vi "MeasurementItems_GetTransferNumber.vi"(8 "error in (no error)":errorcluster, 11 "OXY_SCPI Reseource In":refnum<visa-resource-name>) -> (0 "error out":errorcluster, 1 "communication_data":T1, 2 "Num Transfer Items":i32, 3 "OXY_SCPI Reseource Out":refnum<visa-resource-name>)   [LabVIEW 2018, in "OXYGEN.lvlib"]
doc: "Queries the number of items to be transferred."
uses:
  OXYGEN.lvlib
  TypeDefs/Cluster_RawCommData.ctl
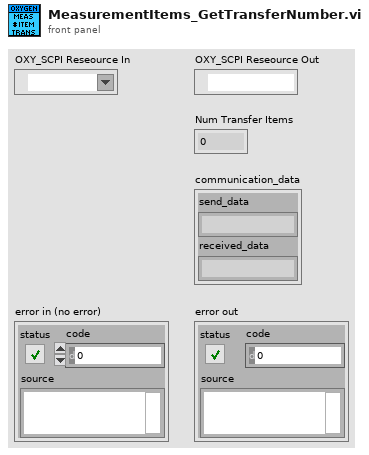
[diagram p1: front panel]
types:
  T1 = typedef "OXYGEN.lvlib/Cluster_RawCommData.ctl" = cluster{"send_data":string, "received_data":string}
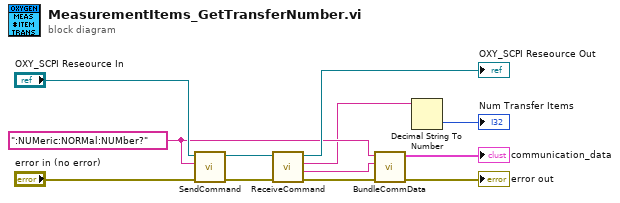
[diagram p0: block diagram]
diagram:
  w4 = ":NUMeric:NORMal:NUMber?" ("String to Send")
  n1 = call "SendCommand.vi"("error in (no error)"="error in (no error)", "String to Send"=w4, "OXY_SCPI Reseource In"="OXY_SCPI Reseource In") -> ("error out"=w12:errorcluster, "OXY_SCPI Reseource Out"=w11:refnum<visa-resource-name>)  [unwired: 7 in]
  n2 = call "ReceiveCommand.vi"("error in (no error)"=w12, "OXY_SCPI Reseource In"=w11) -> ("error out"=w7:errorcluster, "received Data with Header"=w5:string, "received Data"=w2:string, "OXY_SCPI Reseource Out"=→"OXY_SCPI Reseource Out":refnum<visa-resource-name>)  [unwired: 6 in]
  n3 = call "BundleCommData.vi"("error in (no error)"=w7, "received_data"=w5, "send_data"=w4) -> ("error out"=→"error out":errorcluster, "communication_data"=→"communication_data":T1)  [unwired: 7 in]
  n4 = Decimal String To Number(string=w2) -> (number=→"Num Transfer Items":i32)  [unwired: 2 in, 1 out]
